vi "shorttolongtime.vi"(0 "object in":refnum<class "access_work.lvclass">, 1 "data":string[][](table), 2 "table输入":string(combo), 5 "error in (no error)":errorcluster) -> (14 "object out":refnum<class "access_work.lvclass">, 15 "输出数组":string[][](array[string]), 19 "error out":errorcluster)   [LabVIEW 2016, in "access_work.lvclass"]
uses:
  access_work.lvclass
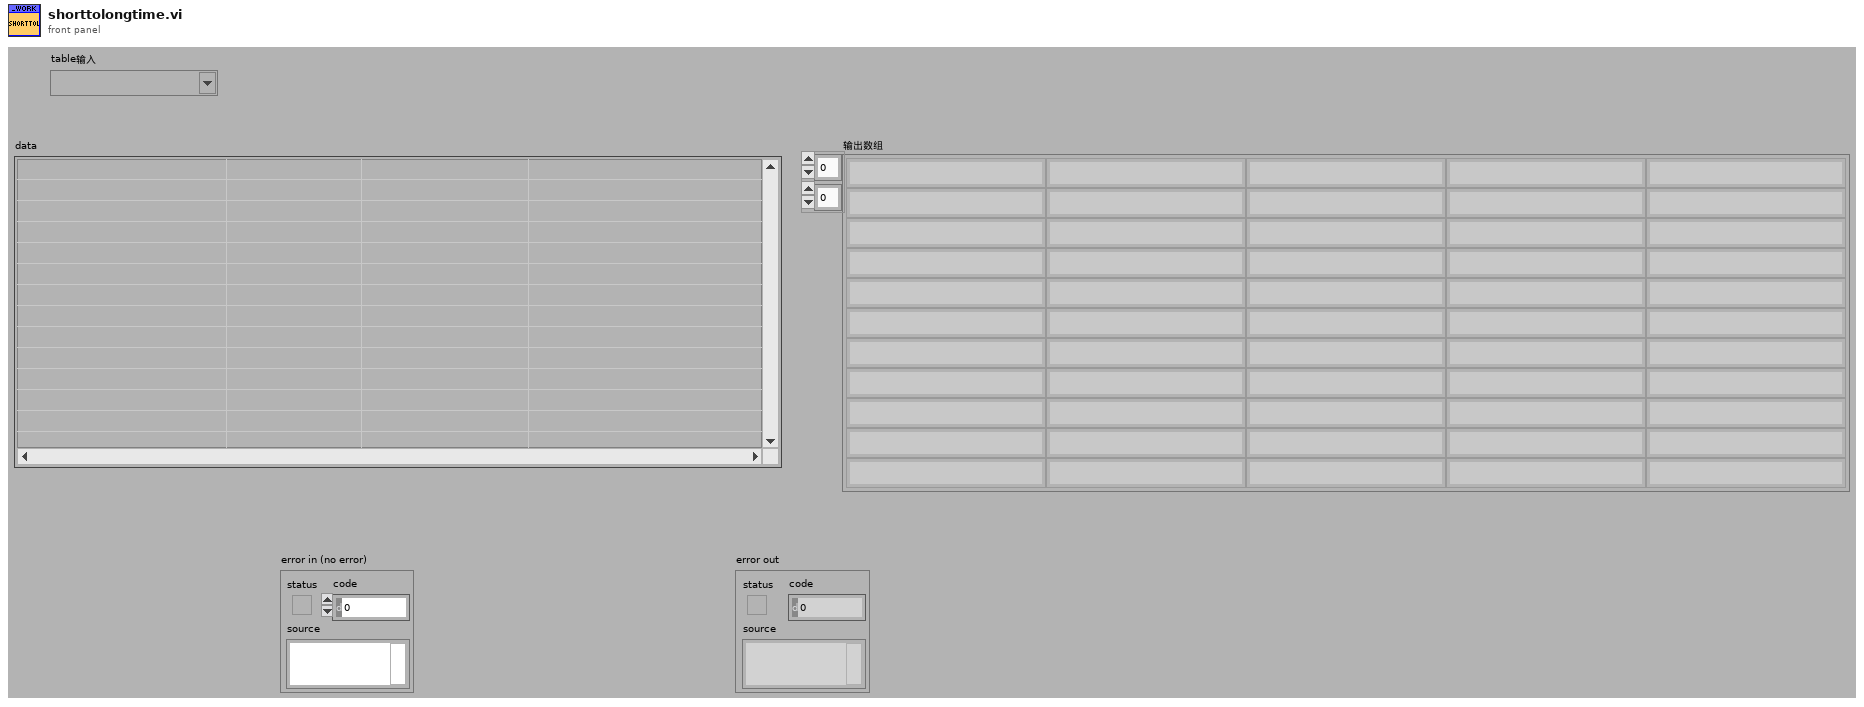
[diagram p1: front panel]
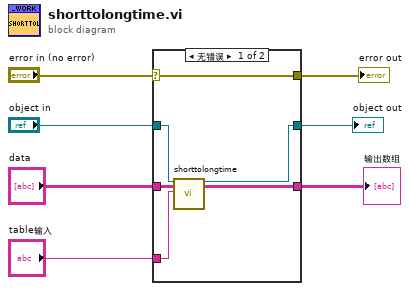
[diagram p0: block diagram]
diagram:
  n1 = case shown="无错误" "error in (no error)" {
    selector: "error in (no error)" -> [w13 w15]
    tunnel: [w13 w15] -> w6
    tunnel: [w8 w14] -> w4
    tunnel: "object in" -> [w12 w14]
    tunnel: "data" -> [w11 _]
    tunnel: "table输入" -> [w10 _]
    tunnel: [w9 _] -> w1
    frame No Error {
      n2 = call-dynamic "shorttolongtime.vi"("object in"=w12, "data"=w11, "table输入"=w10) -> ("object out"=w8:refnum<class "access_work.lvclass">, "输出数组"=w9:string[][])  [unwired: 14 in, 1 out]
    }
    frame Error {
    }
  }
  "error out" <- w6
  "object out" <- w4
  "输出数组" <- w1
